vi "Get Elevator Direction.vi"(8 "error in (no error)":errorcluster, 10 "Elevator Direction":T1, 11 "Elevator Controller in":refnum<class "Elevator Controller.lvclass">) -> (0 "error out":errorcluster, 3 "Elevator Controller out":refnum<class "Elevator Controller.lvclass">)   [LabVIEW 2019, in "Elevator Controller.lvlib" / "Elevator Controller.lvclass"]
uses:
  Elevator Controller.lvclass
  Sim Display Console Actor/Elevator Controller/Elevator Direction.ctl
  Elevator Controller.lvclass/Elevator Controller.ctl
  Sim Display Console Actor/Elevator Controller/Sim Display Console Actor.lvclass
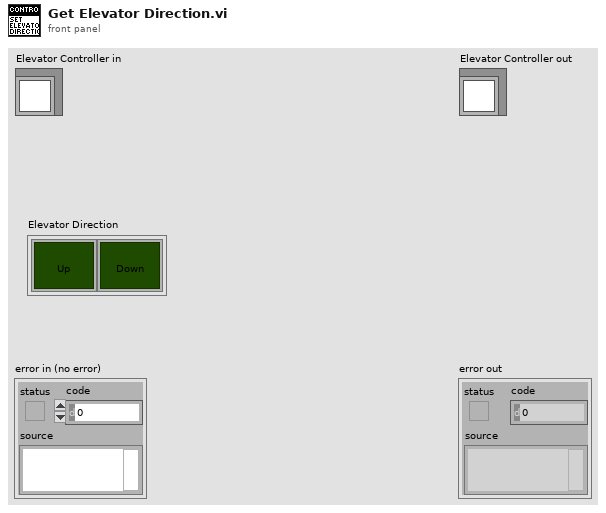
[diagram p1: front panel]
types:
  T1 = typedef "Sim Display Console Actor.lvlib/Sim Display Console Actor.lvclass/Elevator Direction.ctl" = cluster{"Open Door":bool, "Close Door":bool}
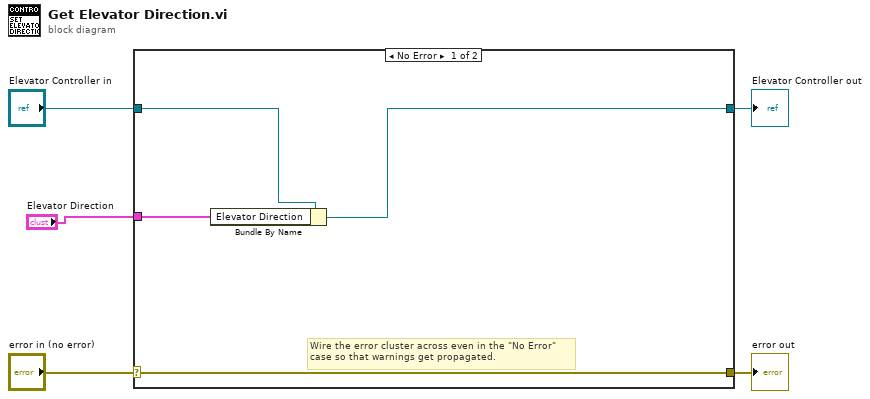
[diagram p0: block diagram]
diagram:
  n1 = case shown="No Error" "error in (no error)" {
    selector: "error in (no error)" -> [w9 w11]
    tunnel: [w9 w11] -> w4
    tunnel: [w6 w10] -> w2
    tunnel: "Elevator Controller in" -> [w8 w10]
    tunnel: "Elevator Direction" -> [w7 _]
    frame No Error {
      # "Wire the error cluster across even in the \"No Error\"\ncase so that warnings get propagated."
      n2 = Bundle By Name(cluster=w8, "Elevator Direction"=w7) -> (w6:refnum<class "Elevator Controller.lvclass">)
    }
    frame Error {
    }
  }
  "error out" <- w4
  "Elevator Controller out" <- w2
